vi "handleTimeout.vi"(8 "error in (no error)":errorcluster, 9 "samples":dbl format="%#_13g", 10 "kickForceArray in":dbl[][](array[numeric]), 11 "Game in":refnum<class "Game.lvclass">) -> (0 "error out":errorcluster, 1 "nextState":T1, 2 "kickForceArrayWithCurrentSampleDeleted":dbl[][](array[numeric]), 3 "Game out":refnum<class "Game.lvclass">)   [LabVIEW 2020, in "Game.lvclass"]
uses:
  Game.lvclass
  Controls/KickForceEnum.ctl
  Utilities_class/Utilities.lvclass
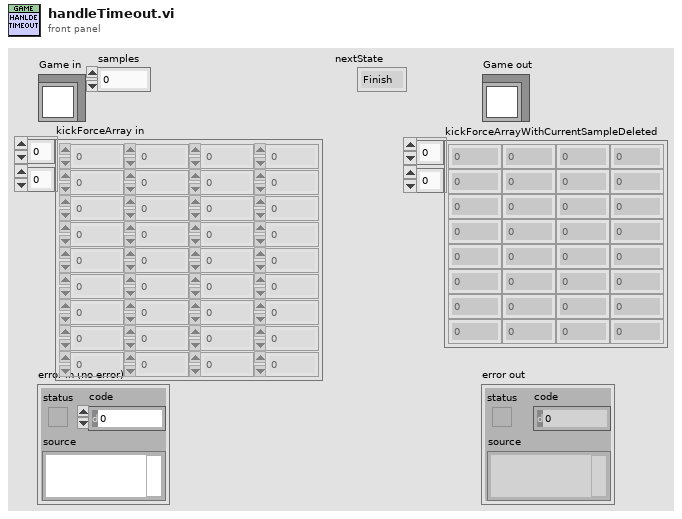
[diagram p1: front panel]
types:
  T1 = typedef "KickForceEnum.ctl" = enum16{"Finish", "GoToNextKickForce", "WaitBall", "KickBall", "ReplaceBall"}
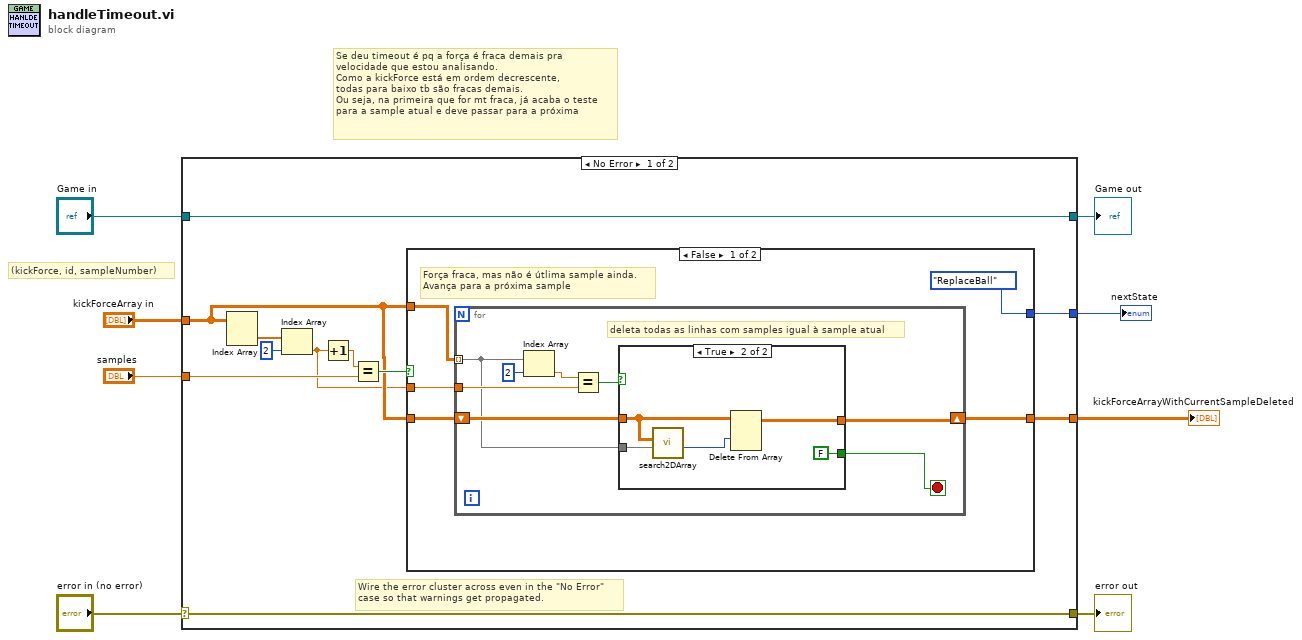
[diagram p0: block diagram]
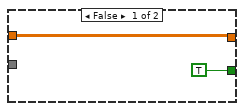
[diagram p2: hidden frame]
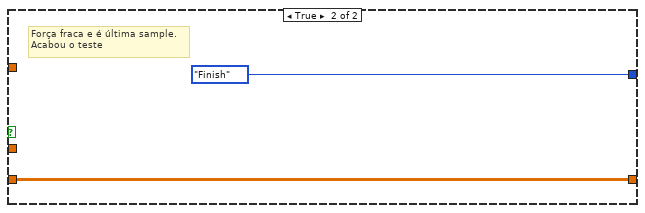
[diagram p3: hidden frame]
diagram:
  # "Se deu timeout é pq a força é fraca demais pra\nvelocidade que estou analisando.\nComo a kickForce está em ordem decrescente,\ntodas para baixo tb são fracas demais.\nOu seja, na primeira que for mt fraca, já acaba o teste\npara a sample atual e deve passar para a próxima"
  # "(kickForce, id, sampleNumber)"
  n1 = case shown="No Error" "error in (no error)" {
    selector: "error in (no error)" -> [w18 w43]
    tunnel: [w18 w43] -> w7
    tunnel: [w19 w42] -> w5
    tunnel: "Game in" -> [w19 w42]
    tunnel: "kickForceArray in" -> [w11 _]
    tunnel: "samples" -> [w14 _]
    tunnel: [w12 _] -> w2
    tunnel: [w9 _] -> w1
    frame No Error {
      # "Wire the error cluster across even in the \"No Error\"\ncase so that warnings get propagated."
      n2 = Index Array(array=w11) -> (element=w17:dbl[])  [unwired: 2 in]
      n3 = Index Array(array=w17, index=2) -> (element=w10:dbl)
      n4 = Increment(x=w10) -> (x+1=w15:dbl)
      n5 = Equal?(x=w15, y=w14) -> (x = y?=w13:bool)
      n6 = case shown="False" w13 {
        tunnel: [KickForceEnum."ReplaceBall" ("Enum 2") KickForceEnum."Finish" ("Enum 2")] -> w12
        tunnel: w11 -> [w23 _]
        tunnel: w11 -> [w22 w40]
        tunnel: w10 -> [w21 _]
        tunnel: [w20 w40] -> w9
        frame False {
          # "Força fraca, mas não é útlima sample ainda.\nAvança para a próxima sample"
          n7 = for {
            tunnel: w23 -> [w25] mode=indexing
            shift-right: [w29] -> w20
            shift-left: w22 -> [w26]
            tunnel: w21 -> [w30]
            stop <- w27 stop-if-true
            # "deleta todas as linhas com samples igual à sample atual"
            n8 = Index Array(array=w25, index=2) -> (element=w31:dbl)
            n9 = Equal?(x=w31, y=w30) -> (x = y?=w28:bool)
            n10 = case shown="True" w28 {
              tunnel: w26 -> [w34 w37]
              tunnel: [w34 w39] -> w29
              tunnel: [TRUE FALSE] -> w27
              tunnel: w25 -> [_ w36]
              frame False {
              }
              frame True {
                n11 = call "search2DArray.vi"("1DArrayToBeSearched"=w36, "2DArray"=w37) -> ("firstIndexOfSearched1DArray"=w35:i32)  [unwired: 6 in, 3 out]
                n12 = Delete From Array(array=w37, index (row)=w35) -> (array with subset deleted=w39:dbl[][])  [unwired: 2 in, 1 out]
              }
            }
          }
        }
        frame True {
          # "Força fraca e é última sample.\nAcabou o teste"
        }
      }
    }
    frame Error {
    }
  }
  "error out" <- w7
  "Game out" <- w5
  "nextState" <- w2
  "kickForceArrayWithCurrentSampleDeleted" <- w1
